vi "Apend Assertion Result to Case Element.vi"(8 "error in (no error)":errorcluster, 9 "Assertion Result":T1={"Status"=enum."Passed", "Message"="", "Description"="", "Assertion Type"=enum."None"}, 10 "Test Case Element in":refnum<k20>, 11 "XML Report In":refnum<class "XML Report.lvclass">) -> (0 "error out":errorcluster, 2 "Test Case Element out":refnum<k20>, 3 "XML Report Out":refnum<class "XML Report.lvclass">)   [LabVIEW 2020, in "XML Report.lvclass"]
uses:
  XML Report.lvclass
  Result Types/Assertion Result/Assertion Result.ctl
  Rewrite Project/Result/Status.ctl
  Result Types/Assertion Result/Public/TypeDefs/Assertion Type.ctl
  XML Report.lvclass/XML Report.ctl
  <vilib>/xml/Close Reference(Node).vi
  <resource>/objmgr/DOMUserDefRef.rc
  <vilib>/xml/NI_XML.lvlib
  Result Types/Assertion Result/Assertion Result.lvlib
  Rewrite Project/Result/Result.lvlib
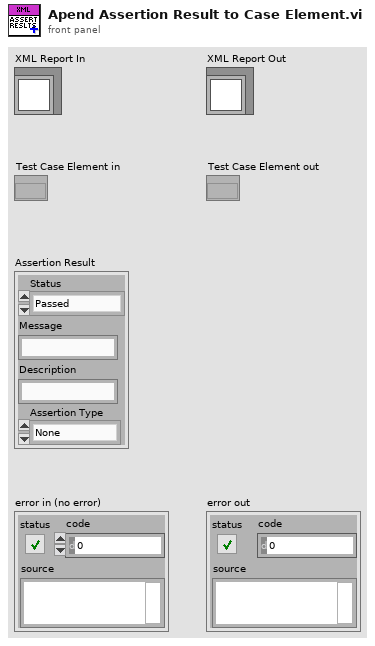
[diagram p1: front panel]
types:
  T1 = typedef "Assertion Result.lvlib/Assertion Result.ctl" = cluster{"Status":T2, "Message":string, "Description":string, "Assertion Type":T3}
  T2 = typedef "Result.lvlib/Status.ctl" = enum16{"", "Passed", "Failed", "Error", "Skipped", "Setup Error", "Broken", "Teardown Error"}
  T3 = typedef "Result.lvlib/Assertion Type.ctl" = enum16{"None", "Pass", "Fail", "Skip", "Pass if Equal", "Fail if Equal", "Pass if Error", "Fail if Error", "Pass if", "Fail if"}
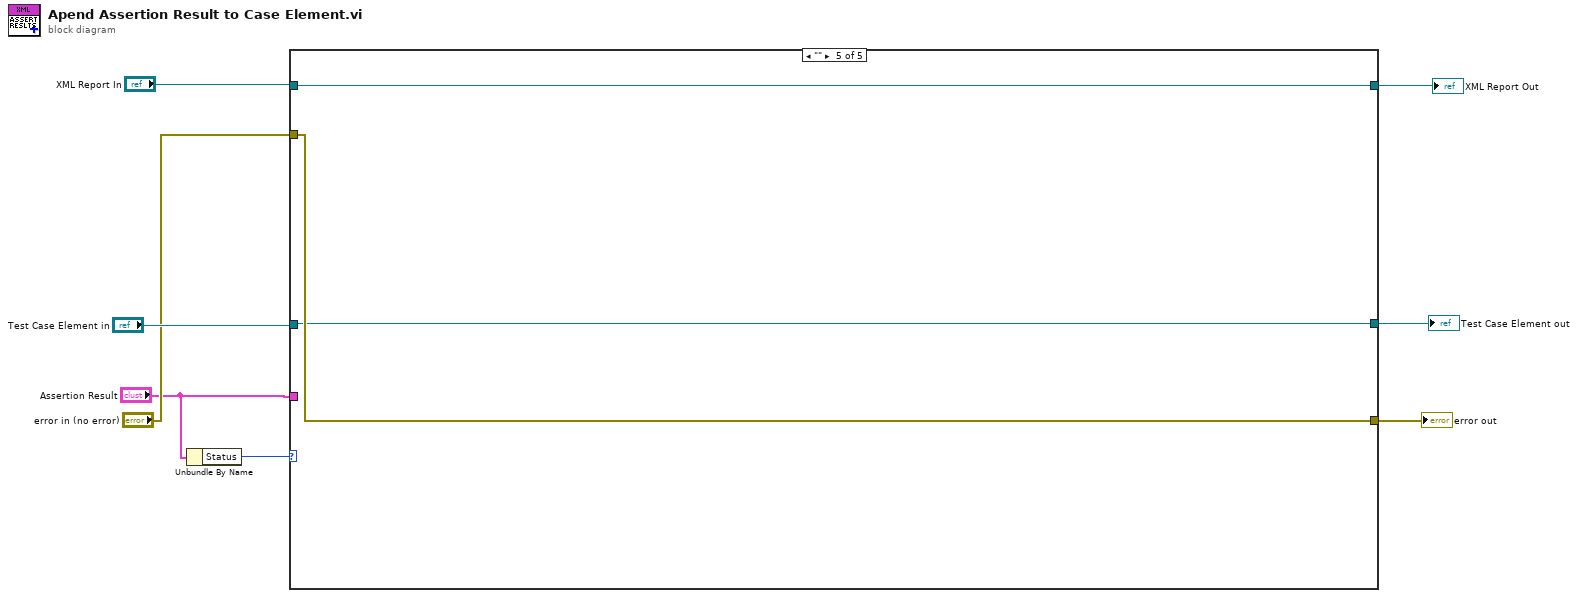
[diagram p0: block diagram]
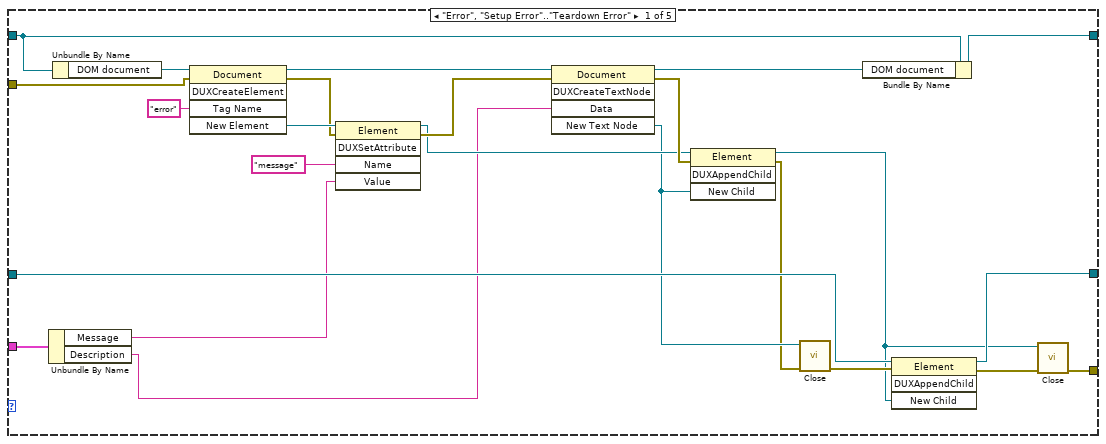
[diagram p2: hidden frame]
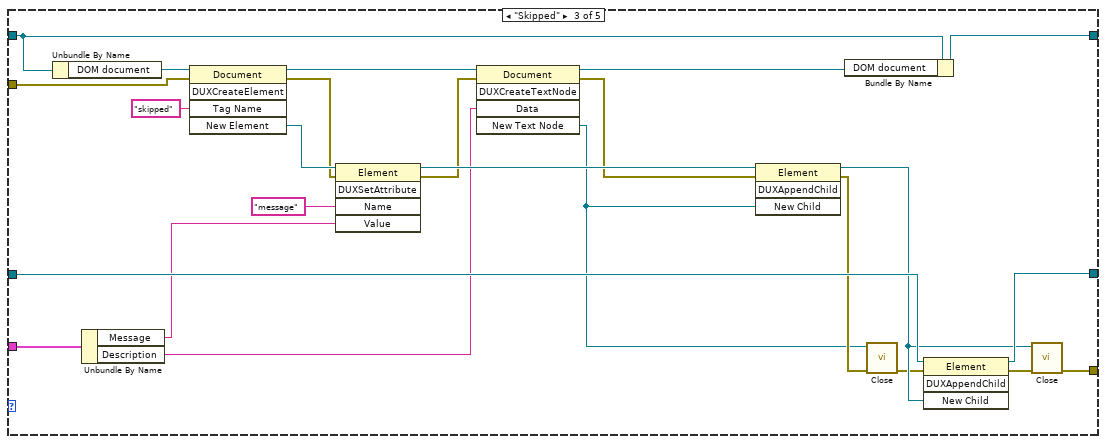
[diagram p4: hidden frame]
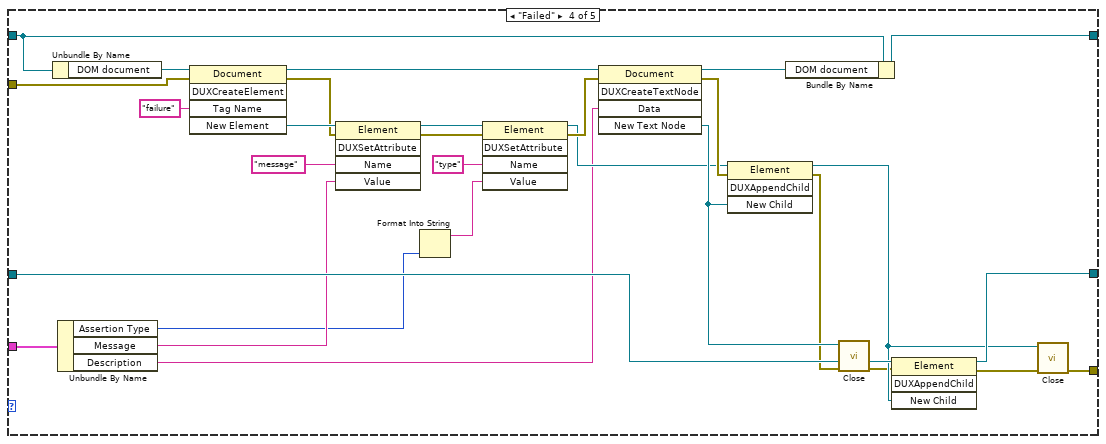
[diagram p5: hidden frame]
diagram:
  n1 = Unbundle By Name("Assertion Result") -> ("Status"=w2:T2)
  n2 = case shown="\"\"" w2 {
    tunnel: "XML Report In" -> [w31 w35 w58 w87 w91]
    tunnel: [w32 w35 w59 w88 w91] -> w8
    tunnel: "Assertion Result" -> [w11 _ w38 w63 _]
    tunnel: "Test Case Element in" -> [w25 w34 w51 w74 w89]
    tunnel: [w24 w34 w50 w75 w89] -> w5
    tunnel: [w22 w33 w47 w76 w90] -> w4
    tunnel: "error in (no error)" -> [w12 w33 w39 w64 w90]
    frame "Error", "Setup Error".."Teardown Error" {
      n3 = Unbundle By Name(w11) -> ("Message"=w10:string, "Description"=w9:string)
      n4 = Unbundle By Name(w31) -> ("DOM document"=w30:refnum<k20>)
      n5 = invoke class="Document" method="DUXCreateElement"(reference=w30, error in=w12, "Tag Name"="error") -> (reference out=w19:refnum<k20>, error out=w27:errorcluster, "New Element"=w28:refnum<k20>)  [unwired: 2 in, 2 out]
      n6 = invoke class="Element" method="DUXSetAttribute"(reference=w28, error in=w27, "Name"="message", "Value"=w10) -> (reference out=w17:refnum<k20>, error out=w20:errorcluster)  [unwired: 1 in, 3 out]
      n7 = invoke class="Document" method="DUXCreateTextNode"(reference=w19, error in=w20, "Data"=w9) -> (reference out=w18:refnum<k20>, error out=w21:errorcluster, "New Text Node"=w16:refnum<k20>)  [unwired: 2 in, 2 out]
      n8 = invoke class="Element" method="DUXAppendChild"(reference=w17, error in=w21, "New Child"=w16) -> (reference out=w13:refnum<k20>, error out=w15:errorcluster)  [unwired: 1 in, 2 out]
      n9 = call-poly <vilib>:"Close.vi"("error in (no error)"=w15, "node"=w16) -> ("error out"=w14:errorcluster)  [unwired: 7 in]
      n10 = Bundle By Name(cluster=w31, "DOM document"=w18) -> (w32:refnum<class "XML Report.lvclass">)
      n11 = invoke class="Element" method="DUXAppendChild"(reference=w25, error in=w14, "New Child"=w13) -> (reference out=w24:refnum<k20>, error out=w23:errorcluster)  [unwired: 1 in, 2 out]
      n12 = call-poly <vilib>:"Close.vi"("error in (no error)"=w23, "node"=w13) -> ("error out"=w22:errorcluster)  [unwired: 7 in]
    }
    frame "Passed" {
    }
    frame "Skipped" {
      n13 = Unbundle By Name(w58) -> ("DOM document"=w57:refnum<k20>)
      n14 = Unbundle By Name(w38) -> ("Message"=w37:string, "Description"=w36:string)
      n15 = invoke class="Document" method="DUXCreateElement"(reference=w57, error in=w39, "Tag Name"="skipped") -> (reference out=w46:refnum<k20>, error out=w54:errorcluster, "New Element"=w55:refnum<k20>)  [unwired: 2 in, 2 out]
      n16 = invoke class="Element" method="DUXSetAttribute"(reference=w55, error in=w54, "Name"="message", "Value"=w37) -> (reference out=w52:refnum<k20>, error out=w45:errorcluster)  [unwired: 1 in, 3 out]
      n17 = invoke class="Document" method="DUXCreateTextNode"(reference=w46, error in=w45, "Data"=w36) -> (reference out=w43:refnum<k20>, error out=w44:errorcluster, "New Text Node"=w40:refnum<k20>)  [unwired: 2 in, 2 out]
      n18 = invoke class="Element" method="DUXAppendChild"(reference=w52, error in=w44, "New Child"=w40) -> (reference out=w49:refnum<k20>, error out=w42:errorcluster)  [unwired: 1 in, 2 out]
      n19 = Bundle By Name(cluster=w58, "DOM document"=w43) -> (w59:refnum<class "XML Report.lvclass">)
      n20 = call-poly <vilib>:"Close.vi"("error in (no error)"=w42, "node"=w40) -> ("error out"=w41:errorcluster)  [unwired: 7 in]
      n21 = invoke class="Element" method="DUXAppendChild"(reference=w51, error in=w41, "New Child"=w49) -> (reference out=w50:refnum<k20>, error out=w48:errorcluster)  [unwired: 1 in, 2 out]
      n22 = call-poly <vilib>:"Close.vi"("error in (no error)"=w48, "node"=w49) -> ("error out"=w47:errorcluster)  [unwired: 7 in]
    }
    frame "Failed" {
      n23 = Unbundle By Name(w87) -> ("DOM document"=w86:refnum<k20>)
      n24 = Unbundle By Name(w63) -> ("Assertion Type"=w61:T3, "Message"=w62:string, "Description"=w60:string)
      n25 = invoke class="Document" method="DUXCreateElement"(reference=w86, error in=w64, "Tag Name"="failure") -> (reference out=w71:refnum<k20>, error out=w83:errorcluster, "New Element"=w84:refnum<k20>)  [unwired: 2 in, 2 out]
      n26 = invoke class="Element" method="DUXSetAttribute"(reference=w84, error in=w83, "Name"="message", "Value"=w62) -> (reference out=w81:refnum<k20>, error out=w80:errorcluster)  [unwired: 1 in, 3 out]
      n27 = Format Into String(w61) -> (resulting string=w78:string)  [unwired: 3 in, 1 out]
      n28 = invoke class="Element" method="DUXSetAttribute"(reference=w81, error in=w80, "Name"="type", "Value"=w78) -> (reference out=w68:refnum<k20>, error out=w70:errorcluster)  [unwired: 1 in, 3 out]
      n29 = invoke class="Document" method="DUXCreateTextNode"(reference=w71, error in=w70, "Data"=w60) -> (reference out=w72:refnum<k20>, error out=w73:errorcluster, "New Text Node"=w69:refnum<k20>)  [unwired: 2 in, 2 out]
      n30 = invoke class="Element" method="DUXAppendChild"(reference=w68, error in=w73, "New Child"=w69) -> (reference out=w67:refnum<k20>, error out=w66:errorcluster)  [unwired: 1 in, 2 out]
      n31 = Bundle By Name(cluster=w87, "DOM document"=w72) -> (w88:refnum<class "XML Report.lvclass">)
      n32 = call-poly <vilib>:"Close.vi"("error in (no error)"=w66, "node"=w69) -> ("error out"=w65:errorcluster)  [unwired: 7 in]
      n33 = invoke class="Element" method="DUXAppendChild"(reference=w74, error in=w65, "New Child"=w67) -> (reference out=w75:refnum<k20>, error out=w77:errorcluster)  [unwired: 1 in, 2 out]
      n34 = call-poly <vilib>:"Close.vi"("error in (no error)"=w77, "node"=w67) -> ("error out"=w76:errorcluster)  [unwired: 7 in]
    }
    frame "" {
    }
  }
  "XML Report Out" <- w8
  "error out" <- w4
  "Test Case Element out" <- w5
